vi "Acceleration Sensor-Remote.vi"() -> ()   [LabVIEW 2009]
uses:
  <vilib>/NXT/Block Support/NXT_InputPort.ctl
  <vilib>/NXT/Subs/LVHSConnector.ctl
panel:
  out "Status (boolean)":bool caption="Success?"
  out "NXT dup":T1={"error"={"status"=FALSE, "code"=0, "source"=""}, "address"="", "NXT #"=-1, "Show Error"=TRUE} caption="NXT"
  in  "NXT":T1={"error"={"status"=FALSE, "code"=0, "source"=""}, "address"="", "NXT #"=-1, "Show Error"=TRUE}
  in  "Input Port":T2 items=["Port 1", "Port 2", "Port 3", "Port 4"]
  # "mindsensors.com\nCopyright (c) 2009 by mindsensors.com\nEmail: info (<at>) mindsensors (<dot>) com\n\nThis program is free software. You can redistribute it and/or modify\nit under the terms of the GNU General Public License as published by\nthe Free Software Foundation; version 3 of the License.\nRead the license at: http://www.gnu.org/licenses/gpl.txt"
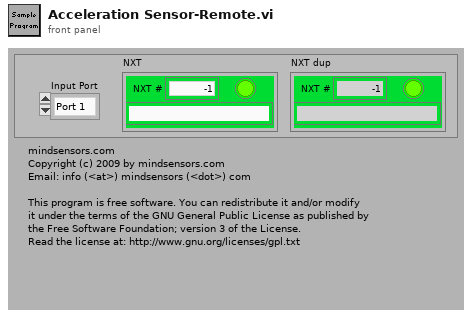
[diagram p1: front panel]
types:
  T1 = typedef "LVHSConnector.ctl" = cluster{"error":errorcluster, "address":string, "NXT #":i32, "Show Error":bool}
  T2 = typedef "NXT_InputPort.ctl" = u8
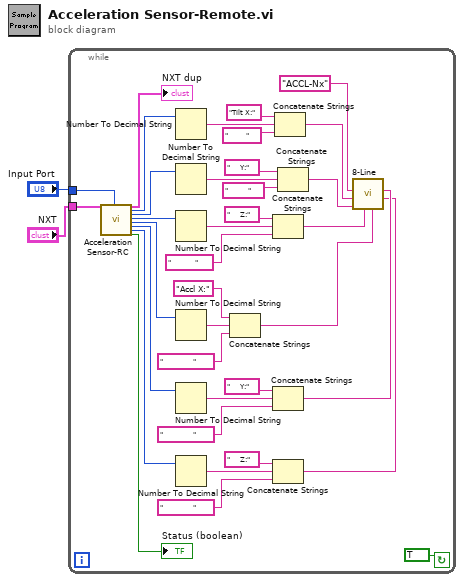
[diagram p0: block diagram]
diagram:
  n1 = while {
    tunnel: "Input Port" -> [w7]
    tunnel: "NXT" -> [w6]
    stop <- TRUE continue-if-true
    n2 = call "Acceleration Sensor-RC.vi"("NXT"=w6, "Input Port"=w7) -> ("NXT dup"=→"NXT dup":T1, "X Tilt"=w4:i16, "Y Tilt"=w22:i16, "Z Tilt"=w21:i16, "X Accel"=w32:i16, "Y Accel"=w27:i16, "Z Accel"=w20:i16, "Status (boolean)"=→"Status (boolean)":bool)  [unwired: 18 in]
    n3 = Number To Decimal String(number=w4) -> (decimal integer string=w36:string)  [unwired: 1 in]
    n4 = Number To Decimal String(number=w22) -> (decimal integer string=w25:string)  [unwired: 1 in]
    n5 = Number To Decimal String(number=w21) -> (decimal integer string=w23:string)  [unwired: 1 in]
    n6 = Number To Decimal String(number=w32) -> (decimal integer string=w33:string)  [unwired: 1 in]
    n7 = Number To Decimal String(number=w27) -> (decimal integer string=w30:string)  [unwired: 1 in]
    n8 = Number To Decimal String(number=w20) -> (decimal integer string=w28:string)  [unwired: 1 in]
    n9 = Concatenate Strings("Accl X:" ("string"), w33, "               " ("string")) -> (w19:string)
    n10 = Concatenate Strings("     Z:" ("string"), w23, "            " ("string")) -> (w15:string)
    n11 = Concatenate Strings("     Y:" ("string"), w30, "               " ("string")) -> (w18:string)
    n12 = Concatenate Strings("     Z:" ("string"), w28, "               " ("string")) -> (w17:string)
    n13 = Concatenate Strings("Tilt X:" ("string"), w36, "         " ("string")) -> (w35:string)
    n14 = Concatenate Strings("     Y:" ("string"), w25, "          " ("string")) -> (w16:string)
    n15 = call "8-Line.vi"("Line 7"=w17, "Line 6"=w18, "Line 5"=w19, "Line 4"=w15, "Line 3"=w16, "Line 2"=w35, "Line 1"="ACCL-Nx") -> ()  [unwired: 4 in, 1 out]
  }
